vi "Prompted Inputs Flatten Test Parameters.vi"(7 "Test Configuration (\"\")":string, 9 "error in (no error)":errorcluster, 10 "Parameter Variant":variant) -> (1 "error out":errorcluster, 2 "Parameter String":string)   [LabVIEW 2011]
uses:
  TypeDefs/PI Test Parameters.ctl
  TypeDefs/PI Measurement Cluster.ctl
  TypeDefs/PI Limit Parameters.ctl
  TypeDefs/PI Limit Definition.ctl
  TypeDefs/PI Limit Comparison.ctl
  Prompted Inputs Version.vi
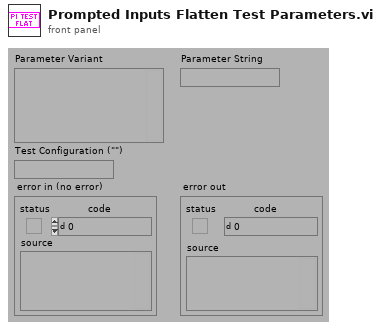
[diagram p1: front panel]
types:
  T1 = typedef "PI Test Parameters.ctl" = cluster{"Measurement":T2, "Limit":T3}
  T2 = typedef "PI Measurement Cluster.ctl" = cluster{"sxFieldId":string, "sValue":string, "nDataType":enum16{"Scalar", "Enumeration"}, "sUnits":string, "sDisplayName":string}
  T3 = typedef "PI Limit Parameters.ctl" = cluster{"Limits On":bool, "Limits":T4[]}
  T4 = typedef "PI Limit Definition.ctl" = cluster{"nComparison":T5, "sValue":string}
  T5 = typedef "PI Limit Comparison.ctl" = enum16{">", ">=", "<", "<=", "<>", "="}
  T6 = typedef "OGAB Version.ctl" = cluster{"Version":string, "Build Number":u32, "Build Date/Time":dbl}
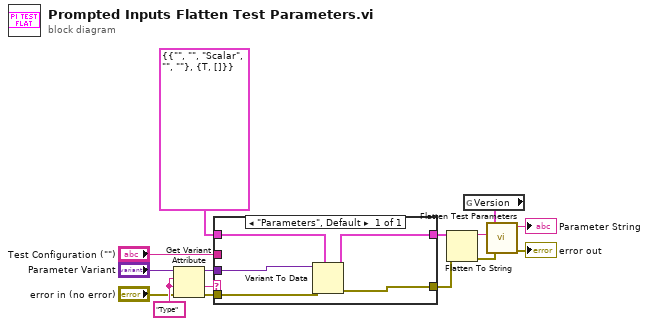
[diagram p0: block diagram]
diagram:
  w14 = "Type" ("name")
  n1 = Get Variant Attribute(Variant="Parameter Variant", name=w14, default value (empty Variant)=w14, error in="error in (no error)") -> (duplicate Variant=w2:variant, value=w1:string, error out=w7:errorcluster)  [unwired: 1 out]
  n2 = case shown="\"Parameters\", Default" w1 {
    tunnel: w2 -> [w20]
    tunnel: T1 {"Measurement"={"sxFieldId"="", "sValue"="", "nDataType"=enum."Scalar", "sUnits"="", "sDisplayName"=""}, "Limit"={"Limits On"=TRUE, "Limits"=[]}} ("Prompted Inputs Test Parameters") -> [w16]
    tunnel: [w17] -> w5
    tunnel: [w19] -> w6
    tunnel: w7 -> [w18]
    tunnel: "Test Configuration (\"\")" -> [_]
    frame "Parameters", Default {
      n3 = Variant To Data(error in=w18, type=w16, Variant=w20) -> (data=w17:T1, error out=w19:errorcluster)
    }
  }
  n4 = Flatten To String(anything=w5, error in (no error)=w6) -> (data string=w13:string, error out=w11:errorcluster)  [unwired: 3 out]
  n5 = global read "Prompted Inputs Version.vi" "Version"() -> (w12:T6)
  n6 = call "Flatten Test Parameters.vi"("error in (no error)"=w11, "Flattened Test Parameters (\"\")"=w13, "Test Version"=w12) -> ("error out"=→"error out":errorcluster, "Flattened Test Parameters with Version"=→"Parameter String":string)  [unwired: 3 out]
